vi "Acquisition Message Loop.vi"(8 "error in (no error)":cluster{"状态":bool, "代码":i32, "源":string} caption="错误输入（无错误）", 9 "数据队列":refnum<queue>, 10 "数据通知器":refnum<notifier>, 11 "消息队列":T1) -> (0 "error out":cluster{"状态":bool, "代码":i32, "源":string} caption="错误输出")   [LabVIEW 2013, in "Acquisition.lvlib"]
doc: "该消息循环负责处理硬件数据采集的相关消息。"
uses:
  Acquisition.lvlib
  support/Message Queue/All Message Queues.ctl
  support/Message Queue/Message Cluster.ctl
  Hardware Configuration.ctl
  Signal Type.ctl
  Acquisition State.ctl
  support/Message Queue/Enqueue Message (Single).vi
  <vilib>/Utility/error.llb/Error Cluster From Error Code.vi
  <vilib>/ErrorRing/Error Ring.xnode
  support/Message Queue/Message Queue.lvlib
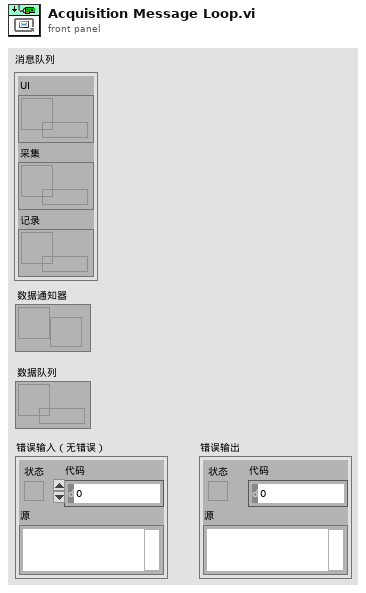
[diagram p1: front panel]
types:
  T1 = typedef "Message Queue.lvlib/All Message Queues.ctl" = cluster{"UI":refnum<queue>, "采集":refnum<queue>, "记录":refnum<queue>}
  T2 = typedef "Acquisition.lvlib/Hardware Configuration.ctl" = cluster{"硬件引用句柄<替换此项>":string, "信号类型<替换该项>":T3}
  T3 = typedef "Acquisition.lvlib/Signal Type.ctl" = enum16{"Sine Wave", "Square with Noise"}
  T4 = typedef "Acquisition.lvlib/Acquisition State.ctl" = enum16{"Idle", "Acquiring"}
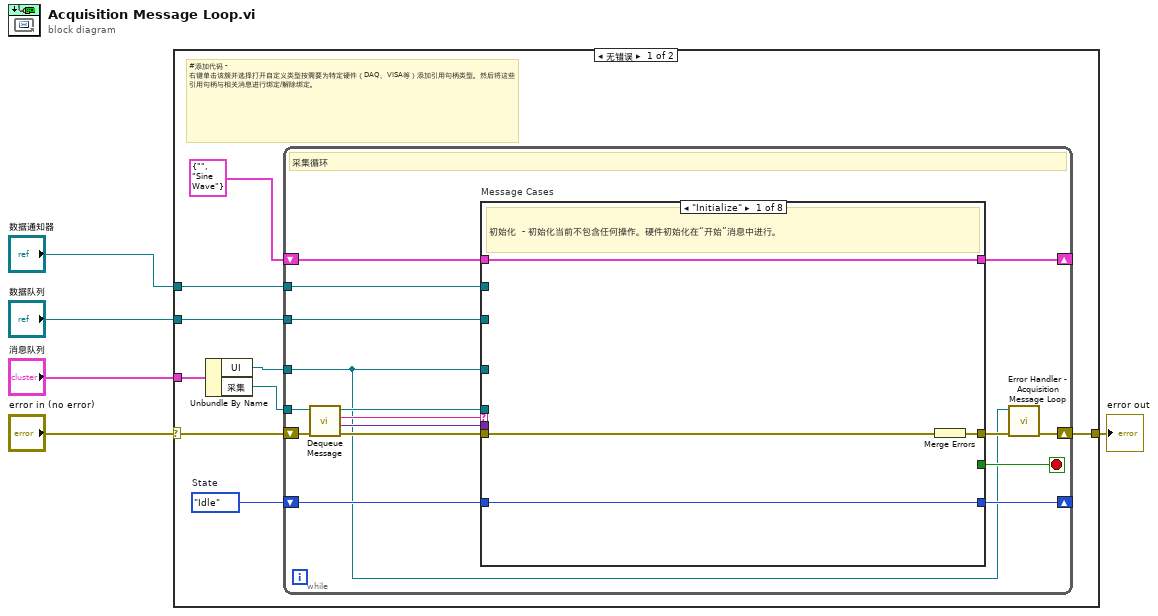
[diagram p0: block diagram]
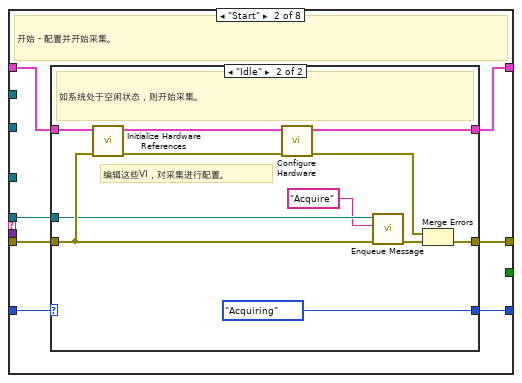
[diagram p2: hidden frame]
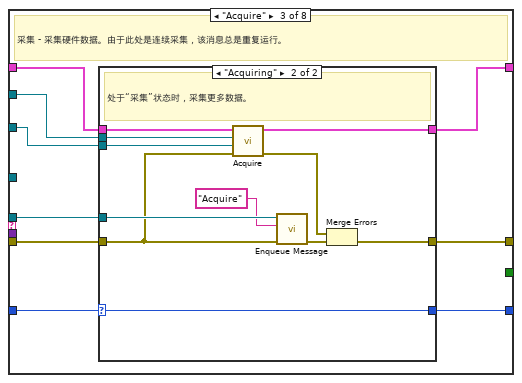
[diagram p4: hidden frame]
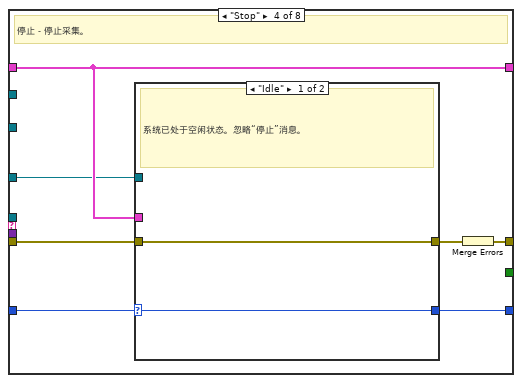
[diagram p6: hidden frame]
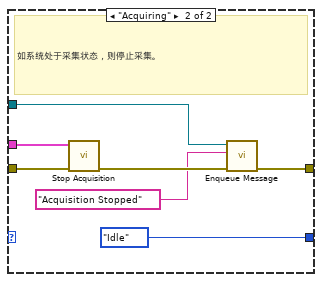
[diagram p7: hidden frame]
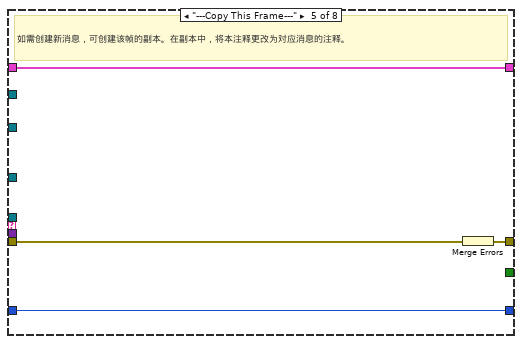
[diagram p8: hidden frame]
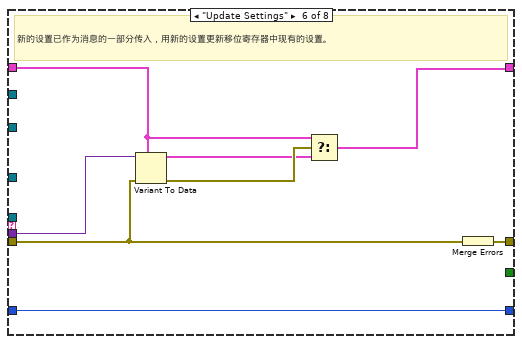
[diagram p9: hidden frame]
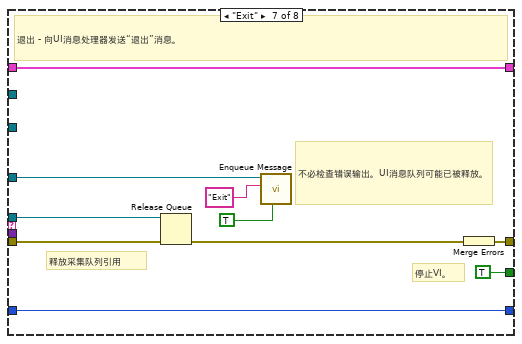
[diagram p10: hidden frame]
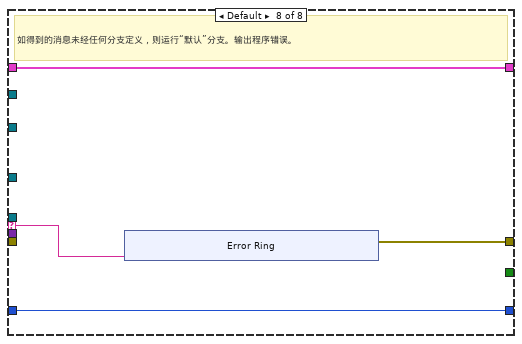
[diagram p11: hidden frame]
diagram:
  n1 = case shown="无错误" "error in (no error)" {
    selector: "error in (no error)" -> [w10 w128]
    tunnel: "消息队列" -> [w14 _]
    tunnel: [w12 w128] -> w4
    tunnel: "数据通知器" -> [w8 _]
    tunnel: "数据队列" -> [w7 _]
    frame No Error {
      w6 = Acquisition_State."Idle"  # State
      # "#添加代码 - 右键单击该簇并选择打开自定义类型按需要为特定硬件（DAQ、VISA等）添加引用句柄类型。然后将这些引用句柄与相关消息进行绑定/解除绑定。"
      n2 = Unbundle By Name(w14) -> ("UI"=w9:refnum<queue>, "采集"=w13:refnum<queue>)
      n3 = while {
        tunnel: w13 -> [w23]
        shift-right: [w29] -> _
        shift-left: T2 {"硬件引用句柄<替换此项>"="", "信号类型<替换该项>"=enum."Sine Wave"} ("Data Cluster") -> [w30]
        shift-right: [w18] -> w12
        shift-left: w10 -> [w27]
        tunnel: w9 -> [w15]
        tunnel: w8 -> [w22]
        tunnel: w7 -> [w21]
        shift-right: [w19] -> _
        shift-left: w6 -> [w20]
        stop <- w28 stop-if-true
        # "采集循环"
        n4 = call "Dequeue Message.vi"("error in (no error)"=w27, "消息队列"=w23) -> ("error out"=w26:cluster{"状态":bool, "代码":i32, "源":string}, "消息数据"=w24:variant, "消息"=w25:string, "消息队列副本"=w16:refnum<queue>)  [unwired: 6 in]
        n5 = case "Message Cases" shown="\"Initialize\"" w25 {
          selector: w25 -> [_ _ _ _ _ _ _ w117]
          tunnel: w16 -> [_ w38 w63 _ _ _ w108 _]
          tunnel: w26 -> [w33 w39 w62 w84 w98 w100 w112 _]
          tunnel: [w34 w41 w64 w85 w96 w106 w115 w118] -> w17
          tunnel: w30 -> [w32 w40 w60 w82 w97 w102 w114 w120]
          tunnel: [w32 w37 w61 w82 w97 w101 w114 w120] -> w29
          tunnel: [_ _ _ _ _ _ TRUE _] -> w28
          tunnel: w24 -> [_ _ _ _ _ w105 _ _]
          tunnel: w15 -> [_ _ _ w79 _ _ w113 _]
          tunnel: w22 -> [_ _ w59 _ _ _ _ _]
          tunnel: w21 -> [_ _ w58 _ _ _ _ _]
          tunnel: w20 -> [w31 w35 w56 w81 w95 w99 w107 w119]
          tunnel: [w31 w36 w57 w80 w95 w99 w107 w119] -> w19
          frame "Initialize" {
            # "初始化  - 初始化当前不包含任何操作。硬件初始化在“开始”消息中进行。"
            n6 = Merge Errors(w33) -> (w34:errorcluster)
          }
          frame "Start" {
            # "开始 - 配置并开始采集。"
            n7 = case shown="\"Idle\"" w35 {
              selector: w35 -> [w42 _]
              tunnel: [w43 w55] -> w41
              tunnel: w40 -> [w44 w54]
              tunnel: w39 -> [w43 w53]
              tunnel: w38 -> [_ w51]
              tunnel: [w44 w47] -> w37
              tunnel: [w42 Acquisition_State."Acquiring" ("Acquisition State")] -> w36
              frame "Acquiring" {
                # "系统已开始采集。忽略“开始”消息。"
              }
              frame "Idle" {
                # "编辑这些VI，对采集进行配置。"
                # "如系统处于空闲状态，则开始采集。"
                n8 = call "Initialize Hardware References.vi"("error in (no error)"=w53, "硬件资源输入"=w54) -> ("error out"=w50:cluster{"状态":bool, "代码":i32, "源":string}, "硬件资源输出"=w48:T2)  [unwired: 8 in]
                n9 = call "Configure Hardware.vi"("error in (no error)"=w50, "硬件资源输入"=w48) -> ("error out"=w49:cluster{"状态":bool, "代码":i32, "源":string}, "硬件资源输出"=w47:T2)  [unwired: 8 in]
                n10 = call-poly "Enqueue Message.vi"("error in (no error)"=w53, "消息"="Acquire" ("Message"), "消息队列"=w51) -> ("error out"=w52:cluster{"状态":bool, "代码":i32, "源":string})  [unwired: 7 in, 1 out]
                n11 = Merge Errors(w49, w52) -> (w55:errorcluster)
              }
            }
          }
          frame "Acquire" {
            # "采集 - 采集硬件数据。由于此处是连续采集，该消息总是重复运行。"
            n12 = case shown="\"Acquiring\"" w56 {
              selector: w56 -> [w65 w69]
              tunnel: [w66 w78] -> w64
              tunnel: w63 -> [_ w76]
              tunnel: w62 -> [w66 w68]
              tunnel: [w67 w74] -> w61
              tunnel: w60 -> [w67 w73]
              tunnel: w59 -> [_ w71]
              tunnel: w58 -> [_ w70]
              tunnel: [w65 w69] -> w57
              frame "Idle" {
                # "如采集处于空闲状态，则忽略“采集”消息。"
              }
              frame "Acquiring" {
                # "处于“采集”状态时，采集更多数据。"
                n13 = call "Acquire.vi"("error in (no error)"=w68, "数据队列"=w70, "数据通知器"=w71, "硬件资源输入"=w73) -> ("error out"=w75:cluster{"状态":bool, "代码":i32, "源":string}, "硬件资源输出"=w74:T2)  [unwired: 6 in]
                n14 = call-poly "Enqueue Message.vi"("error in (no error)"=w68, "消息"="Acquire" ("Message"), "消息队列"=w76) -> ("error out"=w77:cluster{"状态":bool, "代码":i32, "源":string})  [unwired: 7 in, 1 out]
                n15 = Merge Errors(w75, w77) -> (w78:errorcluster)
              }
            }
          }
          frame "Stop" {
            # "停止－停止采集。"
            n16 = case shown="\"Idle\"" w81 {
              selector: w81 -> [w86 _]
              tunnel: w84 -> [w87 w94]
              tunnel: [w87 w90] -> w83
              tunnel: w82 -> [_ w92]
              tunnel: [w86 Acquisition_State."Idle" ("State")] -> w80
              tunnel: w79 -> [_ w89]
              frame "Idle" {
                # "系统已处于空闲状态。忽略“停止”消息。"
              }
              frame "Acquiring" {
                # "如系统处于采集状态，则停止采集。"
                n17 = call "Stop Acquisition.vi"("error in (no error)"=w94, "硬件资源输入"=w92) -> ("error out"=w93:cluster{"状态":bool, "代码":i32, "源":string})  [unwired: 9 in]
                n18 = call-poly "Enqueue Message.vi"("error in (no error)"=w93, "消息"="Acquisition Stopped", "消息队列"=w89) -> ("error out"=w90:cluster{"状态":bool, "代码":i32, "源":string})  [unwired: 7 in, 1 out]
              }
            }
            n19 = Merge Errors(w83) -> (w85:errorcluster)
          }
          frame "---Copy This Frame---" {
            # "如需创建新消息，可创建该帧的副本。在副本中，将本注释更改为对应消息的注释。"
            n20 = Merge Errors(w98) -> (w96:errorcluster)
          }
          frame "Update Settings" {
            # "新的设置已作为消息的一部分传入，用新的设置更新移位寄存器中现有的设置。"
            n21 = Variant To Data(error in=w100, type=w102, Variant=w105) -> (data=w103:T2, error out=w104:errorcluster)
            n22 = Select(t=w102, s=w104, f=w103) -> (s? t:f=w101:T2)
            n23 = Merge Errors(w100) -> (w106:errorcluster)
          }
          frame "Exit" {
            # "不必检查错误输出。UI消息队列可能已被释放。"
            # "释放采集队列引用"
            # "停止VI。"
            # "退出 - 向UI消息处理器发送“退出”消息。"
            n24 = Release Queue(queue=w108, error in (no error)=w112) -> (error out=w109:errorcluster)  [unwired: 1 in, 2 out]
            n25 = call-poly "Enqueue Message.vi"("优先消息？(F)"=TRUE, "消息"="Exit" ("Message"), "消息队列"=w113) -> ()  [unwired: 7 in, 2 out]
            n26 = Merge Errors(w109) -> (w115:errorcluster)
          }
          frame Default {
            # "如得到的消息未经任何分支定义，则运行“默认”分支。输出程序错误。"
            n27 = xnode "Error Ring"("参数 0"=w117) -> ("错误输出"=w118:errorcluster)
          }
        }
        n28 = call "Error Handler - Acquisition Message Loop.vi"("error in (no error)"=w17, "消息队列"=w15) -> ("错误输入副本"=w18:cluster{"状态":bool, "代码":i32, "源":string})  [unwired: 8 in, 1 out]
      }
    }
    frame Error {
    }
  }
  "error out" <- w4
